vi "MO Attributes.vi"(10 "MO Terms":i32[](array[numeric])) -> (1 "Read MO":i32[](array[numeric]), 2 "Init MO":i32[](array[numeric]))   [LabVIEW 2025, in "_Rescript.lvlib" / "Msg.lvlib"]
uses:
  _Rescript/_Rescript.lvclass/_Rescript.ctl
  Msg.lvlib
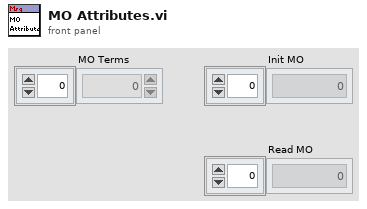
[diagram p1: front panel]
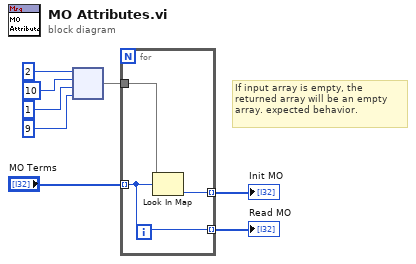
[diagram p0: block diagram]
diagram:
  # "If input array is empty, the returned array will be an empty array. expected behavior."
  n1 = node(2 ("Numeric"), 10 ("Numeric"), 1 ("Numeric"), 9 ("Numeric")) -> (w2:map{i32, i32})
  n2 = for {
    tunnel: [w10] -> w8 mode=indexing
    tunnel: "MO Terms" -> [w9] mode=indexing
    tunnel: w2 -> [w11]
    tunnel: [w9] -> w1 mode=indexing
    n3 = Look In Map(map=w11, key=w9) -> (value=w10:i32)  [unwired: 1 in, 1 out]
  }
  "Init MO" <- w8
  "Read MO" <- w1
